vi "Render.vi"(8 "error in":errorcluster, 10 "Renderer in":refnum<class "Renderer.lvclass">, 11 "Vi in":refnum<class "Vi.lvclass">) -> (0 "error out":errorcluster, 3 "Sections out":refnum<class "Section.lvclass">[](array[class]))   [LabVIEW 2021, in "TAF Proj Document Type.lvlib" / "Vi.lvclass"]
uses:
  <vilib>/Wovalab/AntiDoc/Document Type/Add-ons/LabVIEW TAF Project/Vi/Vi.lvclass
  C:/Program Files (x86)/National Instruments/LabVIEW 2021/vi.lib/Wovalab/AntiDoc/Bloc/Bloc.lvclass
  <vilib>/Wovalab/AntiDoc/Renderer/Renderer.lvclass
  <vilib>/Wovalab/AsciiDoc for LabVIEW/Section/Section.lvclass
  <vilib>/Wovalab/AntiDoc/Document Type/Add-ons/LabVIEW TAF Project/Vi/Vi.lvclass/Vi.ctl
  <vilib>/Wovalab/AntiDoc/Bloc/Bloc.lvclass/Bloc.ctl
  <vilib>/Wovalab/AntiDoc/Renderer/Renderer.lvclass/Renderer.ctl
  <vilib>/Wovalab/AntiDoc/Renderer/Read Image Folder Path.vi
  <vilib>/Wovalab/AntiDoc/Document Type/Add-ons/LabVIEW TAF Project/Vi/Read Conpane Image.vi
  <vilib>/Wovalab/AntiDoc/Bloc/Read Name.vi
  <vilib>/Wovalab/AntiDoc/Document Type/Add-ons/LabVIEW TAF Project/Vi/Read Description.vi
  <vilib>/Wovalab/Asciidoc for LabVIEW/Image/Image.lvclass
  C:/Program Files (x86)/National Instruments/LabVIEW 2021/vi.lib/Wovalab/AsciiDoc for LabVIEW/Adoc-Bloc/Bloc.lvclass
  <vilib>/Wovalab/AsciiDoc for LabVIEW/Paragraph/Paragraph.lvclass
  <vilib>/Wovalab/AsciiDoc for LabVIEW/Section/Add Bloc (array).vi
  <vilib>/Wovalab/AntiDoc/Document Type/Add-ons/LabVIEW TAF Project/TAF Proj Document Type.lvlib
  <vilib>/Wovalab/AntiDoc/Utilities/Utilities.lvlib
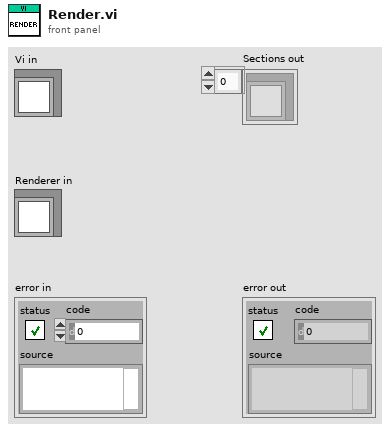
[diagram p1: front panel]
types:
  T1 = typedef "imagedata.ctl" = cluster{"image type":i32, "image depth":i32, "image":u8[], "mask":u8[], "colors":u32[], "Rectangle":cluster{"left":i16, "top":i16, "right":i16, "bottom":i16}}
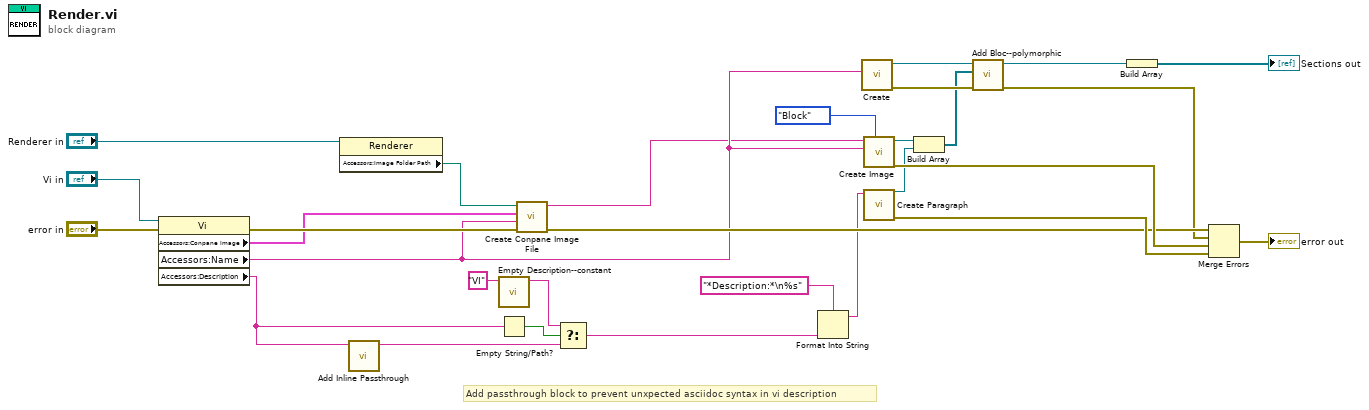
[diagram p0: block diagram]
diagram:
  # "Add passthrough block to prevent unxpected asciidoc syntax in vi description"
  n1 = property class="Vi"(reference="Vi in", error in="error in") -> (error out=w24:errorcluster, "Accessors:Conpane Image"=w14:T1, "Accessors:Name"=w13:string, "Accessors:Description"=w2:string)  [unwired: 1 out]
  n2 = property class="Renderer"(reference="Renderer in") -> ("Accessors:Image Folder Path"=w10:path)  [unwired: 1 in, 2 out]
  n3 = call <vilib>:"Add Inline Passthrough.vi"("String in"=w2) -> ("String out"=w1:string)  [unwired: 10 in]
  n4 = call <vilib>:"Empty Description--constant.vi"("Description Source"="VI") -> ("Empty Description"=w3:string)  [unwired: 10 in]
  n5 = Empty String/Path?(string/path=w2) -> (empty?=w11:bool)
  n6 = call <vilib>:"Create Conpane Image File.vi"("error in"=w24, "Name"=w13, "Conpane Image"=w14, "Image Folder Path"=w10) -> ("error out"=w23:errorcluster, "File Name"=w12:string)  [unwired: 6 in]
  n7 = Select(t=w3, s=w11, f=w1) -> (s? t:f=w8:string)
  n8 = Format Into String(format string="*Description:*\n%s", w8) -> (resulting string=w7:string)  [unwired: 2 in, 1 out]
  n9 = call <vilib>:"Create.vi"("Title"=w13) -> ("error out"=w27:errorcluster, "Section out"=w19:refnum<class "Section.lvclass">)  [unwired: 9 in]
  n10 = call <vilib>:"Create Image.vi"("Type"=enum16{"Block", "Inline"}."Block", "Alt Text"=w13, "Image Path"=w12) -> ("error out"=w26:errorcluster, "Image out"=w16:refnum<class "Image.lvclass">)  [unwired: 7 in]
  n11 = call <vilib>:"Create Paragraph.vi"("Content"=w7) -> ("error out"=w25:errorcluster, "Paragraph out"=w18:refnum<class "Paragraph.lvclass">)  [unwired: 9 in]
  n12 = Build Array(w16, w18) -> (w17:refnum<class "Bloc.lvclass">[])
  n13 = call-poly <vilib>:"Add Bloc--polymorphic.vi"("error in"=w27, "Bloc"=w17, "Section in"=w19) -> ("error out"=w22:errorcluster, "Section out"=w6:refnum<class "Section.lvclass">)  [unwired: 7 in]
  n14 = Build Array(w6) -> (→"Sections out":refnum<class "Section.lvclass">[])
  n15 = Merge Errors(w23, w22, w26, w25) -> (→"error out":errorcluster)
